vi "Fetch Multi Eval Meas Trace ACLR Results.vi"(8 "error in (no error)":errorcluster, 9 "Result Type (Current)":i32(ring) items=["Current", "Average"], 10 "Instance (1)":T2=1, 11 "VISA resource name":refnum<visa-resource-name>) -> (0 "error out":errorcluster, 1 "Trace ACLR Results":T1 {"NR Pos" format="%^.3e"; "Carrier" format="%^.3e"; "NR Neg" format="%^.3e"}, 2 "Reliability":i32, 3 "VISA resource name out":refnum<visa-resource-name>)   [LabVIEW 2015, in "Rohde&Schwarz CMXP NR FR2 Measurement.lvlib"]
doc: "Returns the multi eval measurement ACLR results.\n\nAttributes:\nRSCMXPNRFR2M_ATTR_FETCH_MULTI_EVAL_MEASUREMENT_TRACE_ACLR_AVERAGE_RESULTS\nRSCMXPNRFR2M_ATTR_FETCH_MULTI_EVAL_MEASUREMENT_TRACE_ACLR_CURRENT_RESULTS\n\nRemote-control commands:\nFETCh:NRMMw:MEAS<i>:MEValuation:TRACe:ACLR:AVERage?\nFETCh:NRMMw:MEAS<i>:MEValuation:TRACe:ACLR:CURRent?"
uses:
  <instrlib>/Rohde&Schwarz CMXP NR FR2 Measurement/Rohde&Schwarz CMXP NR FR2 Measurement.lvlib
  <instrlib>/Rohde&Schwarz CMXP NR FR2 Measurement/Private/_Instance.ctl
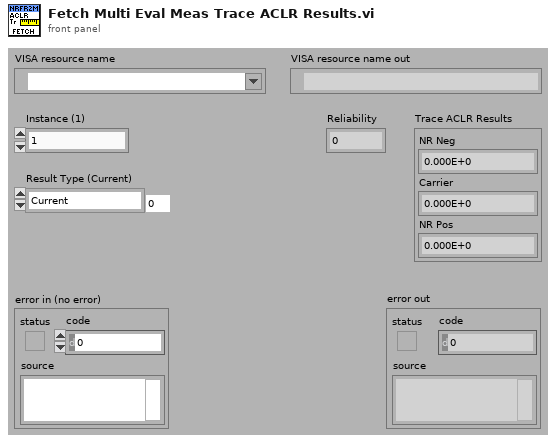
[diagram p1: front panel]
types:
  T1 = cluster{"NR Neg":dbl, "Carrier":dbl, "NR Pos":dbl}
  T2 = typedef "Rohde&Schwarz CMXP NR FR2 Measurement.lvlib/_Instance.ctl" = i32
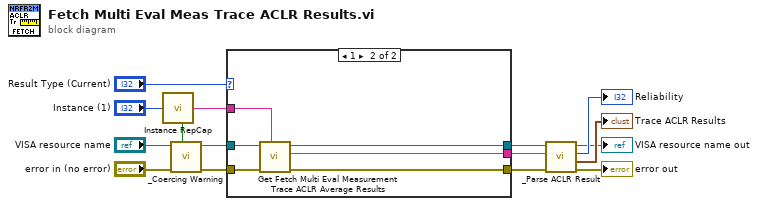
[diagram p0: block diagram]
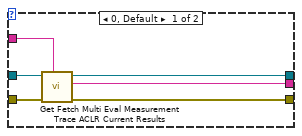
[diagram p2: hidden frame]
diagram:
  n1 = call <instrlib>:"Instance RepCap.vi"("Instance In"="Instance (1)") -> ("In Range?"=w4:bool, "RepCap Identifier Out"=w15:string)  [unwired: 1 in]
  n2 = call <instrlib>:"_Coercing Warning.vi"("In Range?"=w4, "error in (no error)"="error in (no error)", "VISA resource name"="VISA resource name") -> ("error out"=w2:errorcluster, "VISA resource name out"=w3:refnum<visa-resource-name>)  [unwired: 7 in]
  n3 = case shown="1" "Result Type (Current)" {
    tunnel: w2 -> [w20 w27]
    tunnel: w3 -> [w21 w26]
    tunnel: [w17 w25] -> w10
    tunnel: [w18 w24] -> w9
    tunnel: w15 -> [w19 w23]
    tunnel: [w16 w22] -> w14
    frame 0, Default {
      n4 = call "Get Fetch Multi Eval Measurement Trace ACLR Current Results"("Repeated Capabilities"=w19, "error in (no error)"=w20, "instrument handle"=w21) -> ("error out"=w17:errorcluster, "Fetch Multi Eval Measurement Trace ACLR Current Results"=w16:string, "instrument handle out"=w18:refnum<visa-resource-name>)  [unwired: 6 in]
    }
    frame 1 {
      n5 = call "Get Fetch Multi Eval Measurement Trace ACLR Average Results"("Repeated Capabilities"=w23, "error in (no error)"=w27, "instrument handle"=w26) -> ("error out"=w25:errorcluster, "Fetch Multi Eval Measurement Trace ACLR Average Results"=w22:string, "instrument handle out"=w24:refnum<visa-resource-name>)  [unwired: 6 in]
    }
  }
  n6 = call <instrlib>:"_Parse ACLR Result.vi"("error in (no error)"=w10, "Input String"=w14, "VISA resource name"=w9) -> ("error out"=→"error out":errorcluster, "Measurement Result"=→"Trace ACLR Results":T1, "Reliability"=→"Reliability":i32, "VISA resource name out"=→"VISA resource name out":refnum<visa-resource-name>)  [unwired: 5 in]
